vi "Build Rocks.vi"(6 "reference":refnum<vi>, 11 "Input":string) -> (0 "Bottom":i32[](array[numeric]), 1 "Top":i32[](array[numeric]), 2 "Right":i32[](array[numeric]), 3 "Left":i32[](array[numeric]), 4 "reference out":refnum<vi>, 5 "Rocks":cluster{u32[], u32[]})   [LabVIEW 2021, in "d14.lvlib"]
uses:
  d14.lvlib
  <vilib>/Analysis/1siggen.llb/Ramp Pattern by Delta.vi
  <vilib>/Analysis/NI_AALBase.lvlib
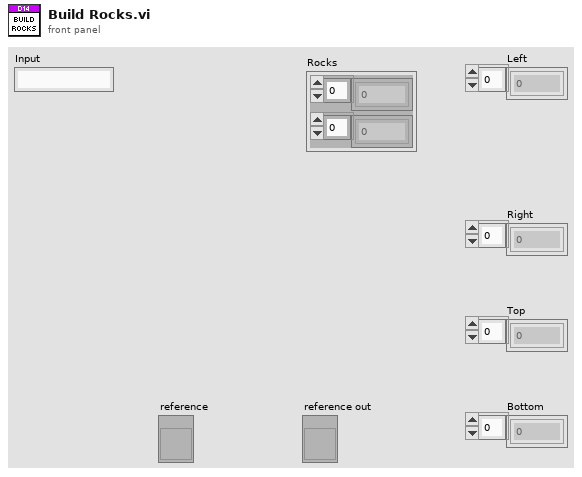
[diagram p1: front panel]
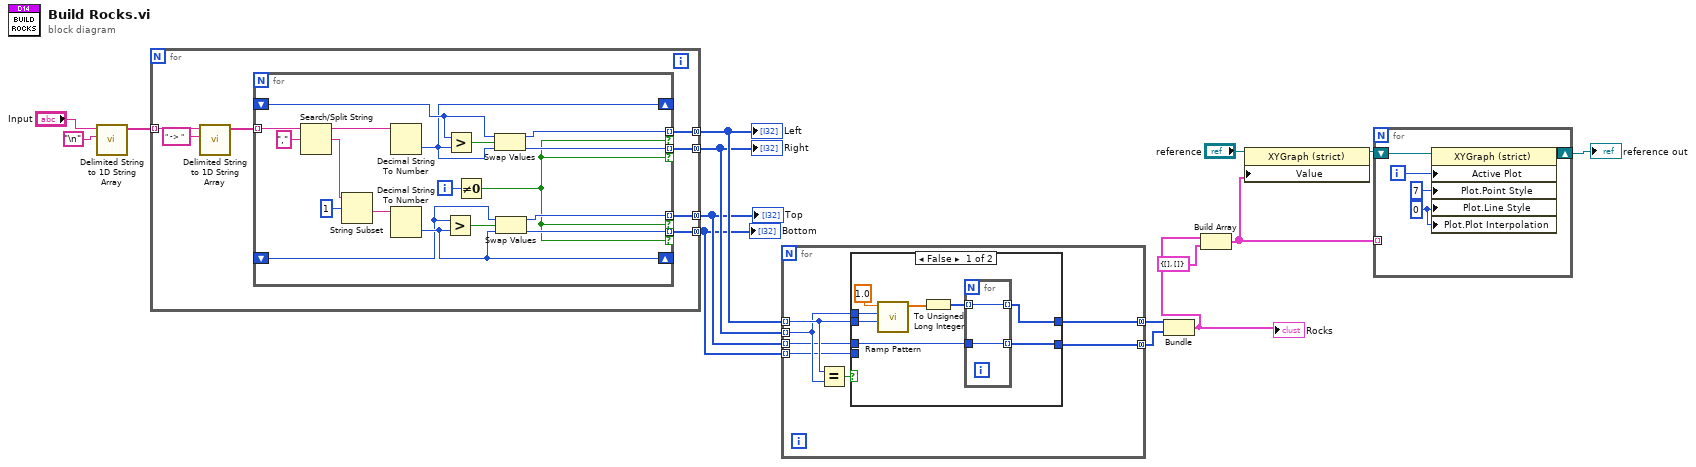
[diagram p0: block diagram]
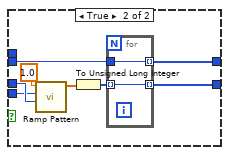
[diagram p2: hidden frame]
diagram:
  n1 = call <vilib>:"Delimited String to 1D String Array.vi"("delimiter"="\n", "delimited string"="Input") -> ("string array"=w15:string[])  [unwired: 9 in]
  n2 = for {
    tunnel: w15 -> [w22] mode=indexing
    tunnel: [w19] -> w12 mode=concatenating
    tunnel: [w18] -> w11 mode=concatenating
    tunnel: [w17] -> w10 mode=concatenating
    tunnel: [w16] -> w9 mode=concatenating
    n3 = call <vilib>:"Delimited String to 1D String Array.vi"("delimiter"=" -> ", "delimited string"=w22) -> ("string array"=w20:string[])  [unwired: 9 in]
    n4 = for {
      tunnel: w20 -> [w40] mode=indexing
      shift-right: [w25] -> _
      shift-left: _ -> [w27]
      tunnel: [w35] -> w19 mode=indexing if=w31
      tunnel: [w34] -> w18 mode=indexing if=w31
      tunnel: [w32] -> w16 mode=indexing if=w31
      shift-right: [w28] -> _
      shift-left: _ -> [w26]
      tunnel: [w33] -> w17 mode=indexing if=w31
      i -> [w36]
      n5 = Search/Split String(string=w40, search string/char (-)=",") -> (substring before match=w37:string, match + rest of string=w38:string)  [unwired: 1 in, 1 out]
      n6 = String Subset(string=w38, offset (0)=1) -> (substring=w24:string)  [unwired: 1 in]
      n7 = Decimal String To Number(string=w37) -> (number=w25:i32)  [unwired: 2 in, 1 out]
      n8 = Decimal String To Number(string=w24) -> (number=w28:i32)  [unwired: 2 in, 1 out]
      n9 = Greater?(x=w26, y=w28) -> (0:w29:bool)
      n10 = Greater?(x=w27, y=w25) -> (0:w30:bool)
      n11 = Not Equal To 0?(x=w36) -> (x != 0?=w31:bool)
      n12 = Swap Values(12:w27, 13:w30, 14:w25) -> (1:w35:i32, 3:w34:i32)
      n13 = Swap Values(12:w26, 13:w29, 14:w28) -> (1:w33:i32, 3:w32:i32)
    }
  }
  "Right" <- w11
  "Bottom" <- w9
  "Top" <- w10
  "Left" <- w12
  n14 = for {
    tunnel: w12 -> [w47] mode=indexing
    tunnel: w11 -> [w46] mode=indexing
    tunnel: w10 -> [w44] mode=indexing
    tunnel: w9 -> [w43] mode=indexing
    tunnel: [w42] -> w3 mode=concatenating
    tunnel: [w41] -> w2 mode=concatenating
    n15 = Equal?(x=w47, y=w46) -> (x = y?=w45:bool)
    n16 = case shown="False" w45 {
      tunnel: w47 -> [w55 w62]
      tunnel: w46 -> [w54 _]
      tunnel: w44 -> [w50 w61]
      tunnel: w43 -> [_ w60]
      tunnel: [w49 w59] -> w42
      tunnel: [w48 w58] -> w41
      frame False {
        n17 = call-poly <vilib>:"Ramp Pattern.vi"("start"=w55, "end"=w54, "delta"=1.0) -> ("Ramp Pattern"=w52:dbl[])  [unwired: 6 in, 2 out]
        n18 = To Unsigned Long Integer(number=w52) -> (unsigned 32bit integer=w51:u32[])
        n19 = for {
          tunnel: w51 -> [w57] mode=indexing
          tunnel: [w57] -> w49 mode=indexing
          tunnel: w50 -> [w56]
          tunnel: [w56] -> w48 mode=indexing
        }
      }
      frame True {
        n20 = call-poly <vilib>:"Ramp Pattern.vi"("start"=w61, "end"=w60, "delta"=1.0) -> ("Ramp Pattern"=w64:dbl[])  [unwired: 6 in, 2 out]
        n21 = To Unsigned Long Integer(number=w64) -> (unsigned 32bit integer=w63:u32[])
        n22 = for {
          tunnel: w63 -> [w67] mode=indexing
          tunnel: [w67] -> w58 mode=indexing
          tunnel: w62 -> [w66]
          tunnel: [w66] -> w59 mode=indexing
        }
      }
    }
  }
  n23 = Bundle(w3, w2) -> (w1:cluster{u32[], u32[]})  [unwired: 1 in]
  "Rocks" <- w1
  n24 = Build Array(w1, cluster{u32[], u32[]} {[], []} ("output cluster")) -> (w4:cluster{u32[], u32[]}[])
  n25 = property on="Property Node" class="XYGraph (strict)"(reference="reference", "Value"=w4) -> (reference out=w7:refnum<vi>)  [unwired: 1 in, 1 out]
  n26 = for {
    shift-right: [w71] -> w5
    shift-left: w7 -> [w72]
    tunnel: w4 -> [_] mode=indexing
    i -> [w70]
    w68 = u8 0 ("Plot.Line Style")
    n27 = property class="XYGraph (strict)"(reference=w72, "Active Plot"=w70, "Plot.Point Style"=u8 7, "Plot.Line Style"=w68, "Plot.Plot Interpolation"=w68) -> (reference out=w71:refnum<vi>)  [unwired: 1 in, 1 out]
  }
  "reference out" <- w5
